vi "CheckInclinometerTimeout.vi"(10 "StateIfNoTimeout":T1, 11 "InclinometerData in":T2) -> (3 "InclinometerData out":T2)   [LabVIEW 2016]
uses:
  InclinometerData.ctl
  InclinometerStates.ctl
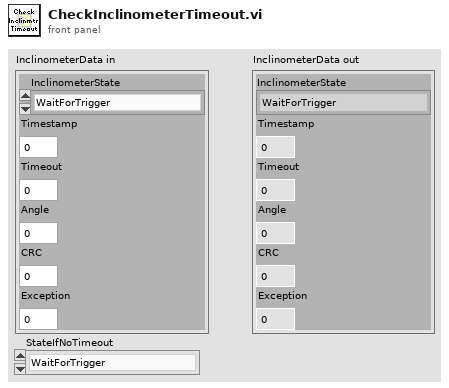
[diagram p1: front panel]
types:
  T1 = typedef "InclinometerStates.ctl" = enum16{"WaitForTrigger", "ClearRxFIFO", "WaitForClearComplete", "WriteAddress", "WriteFunction", "WriteStartAddress1", "WriteStartAddress0", "WriteAddressCount1", "WriteAddressCount0", "WriteCRC1", "WriteCRC0", "ReadAddress", "ReadFunction", "ReadByteCount", "ReadDataByte1", "ReadDataByte0", "ReadDataByte3", "ReadDataByte2", "ReadCRCByte0", "ReadCRCByte1", "CalculateCRC", "ValidateCRC", "MoveTimestamp", "MoveData", "ClearErrorCode", "ReadExceptionCode", "ReadExceptionCRCByte0", "ReadExceptionCRCByte1", "CalculateExceptionCRC", "ValidateExceptionCRC", "ParseExceptionCode", "ResponseAddressError", "ResponseFunctionCodeError", "ResponseByteCountError", "ResponseCRCError", "ResponseUnknownError", "ResponseTimeoutError", "SensorReportsIllegalFunction", "SensorReportsIllegalDataAddress"}
  T2 = typedef "InclinometerData.ctl" = cluster{"InclinometerState":T1, "Timestamp":u64, "Timeout":i32, "Angle":u32, "CRC":u16, "Exception":u8}
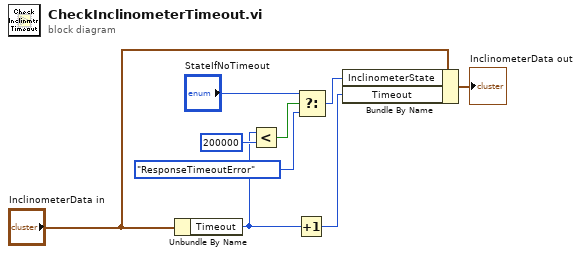
[diagram p0: block diagram]
diagram:
  n1 = Unbundle By Name("InclinometerData in") -> ("Timeout"=w3:i32)
  n2 = Less?(x=w3, y=200000) -> (x < y?=w7:bool)
  n3 = Increment(x=w3) -> (x+1=w9:i32)
  n4 = Select(t="StateIfNoTimeout", s=w7, f=InclinometerStates."ResponseTimeoutError" ("InclinometerState")) -> (s? t:f=w5:T1)
  n5 = Bundle By Name(cluster="InclinometerData in", "InclinometerState"=w5, "Timeout"=w9) -> (→"InclinometerData out":T2)
